vi "抓邊.vi"(0 "Image In":T1, 1 "Process":T7(ring), 2 "Optimized Mode":bool, 3 "Direction":T4(ring), 5 "ROI":T2, 9 "Gap":i32=10 min=1 max=300, 11 "error In":errorcluster, 12 "Edge Options":T5={"Edge Polarity"=0, "Kernel Size"=3, "Width"=3, "Minimum Edge Strength"=10.0, "Interpolation Type"=enum."Bilinear Fixed", "Data Processing Method"=enum."Average"} {"Edge Polarity" items=["All Edges", "Rising Edges", "Falling Edges"]; "Minimum Edge Strength" format="%.2f"; "Width" step=2; "Kernel Size" step=2}, 13 "Point Diameter (5)":u32=5 min=3 max=1000) -> (4 "Image Out":T1, 6 "Line Profile":T3(graph), 10 "Gradient Information":dbl[][](graph), 14 "Line Data":cluster{"X":sgl, "Y":sgl, "T":sgl}, 15 "error out":errorcluster)   [LabVIEW 2015]
uses:
  <vilib>/vision/Measure.llb/Edge Options.ctl
  <vilib>/vision/Measure.llb/Edge Polarity.ctl
  <vilib>/vision/Image Controls.llb/IMAQ Image.ctl
  <vilib>/vision/NI_Vision_Development_Module.lvlib
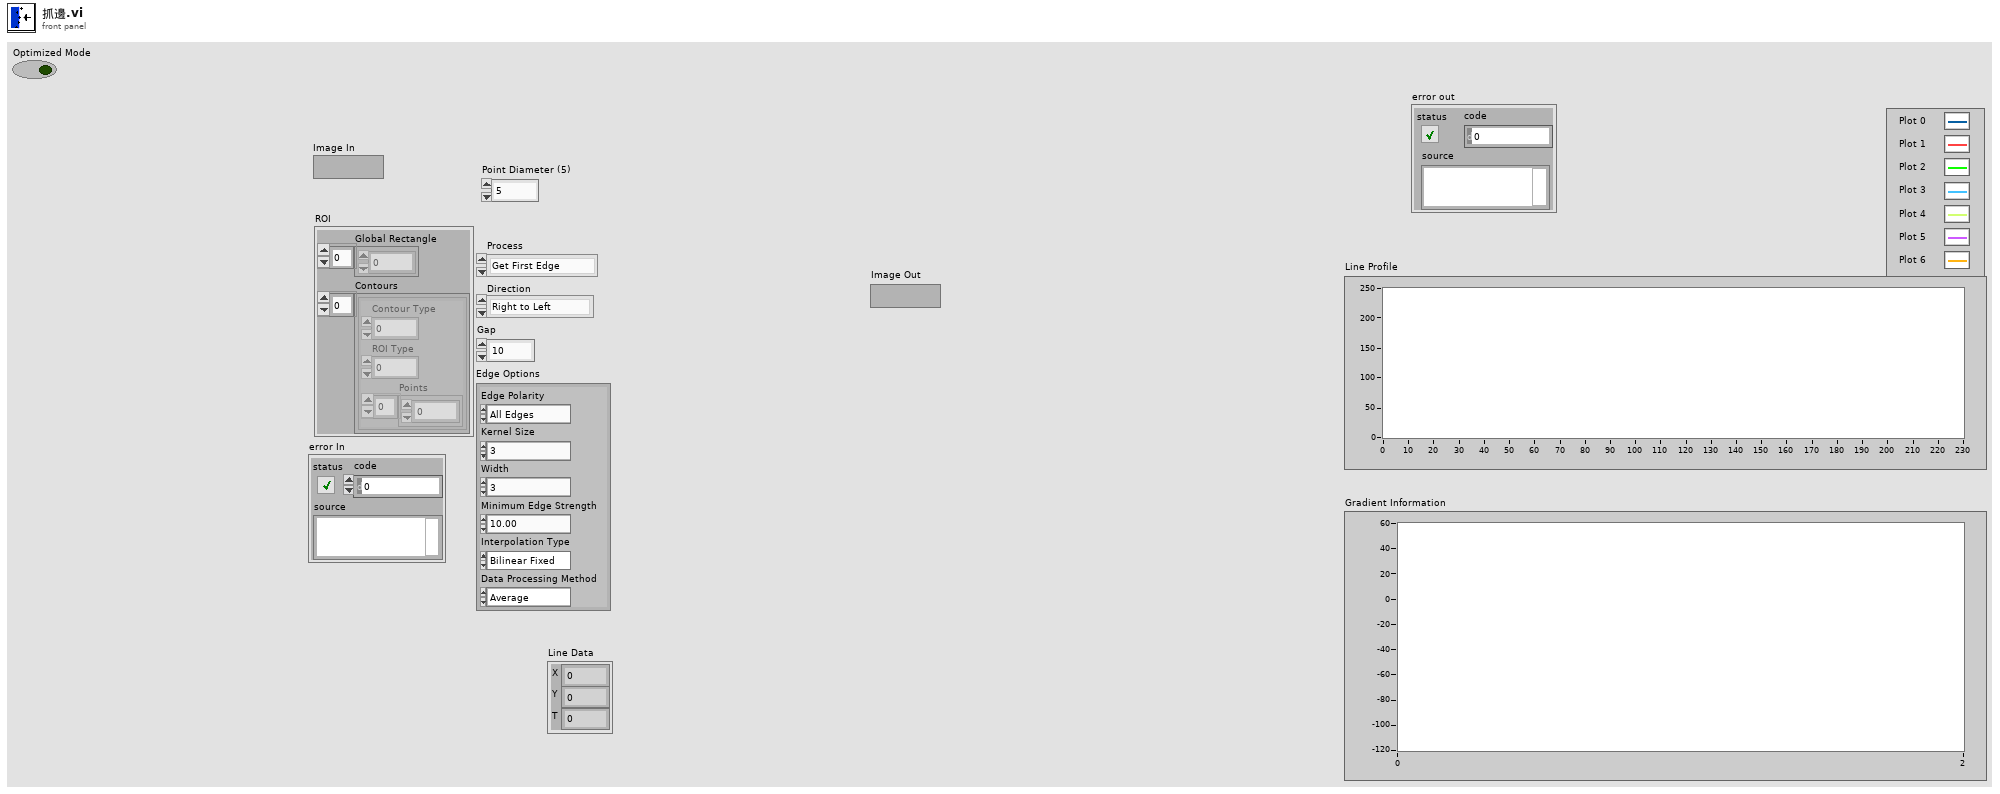
[diagram p1: front panel]
types:
  T1 = typedef "IMAQ Image.ctl" = refnum<image>
  T2 = cluster{"Global Rectangle":i32[], "Contours":cluster{"Contour Type":u32, "ROI Type":u32, "Points":i32[]}[]}
  T3 = cluster{"x0":sgl, "dx":sgl, "Pixels Line":sgl[]}[]
  T4 = enum16{"Right to Left", "Left  to Right", "Up to Down", "Down to Up"}
  T5 = typedef "Edge Options.ctl" = cluster{"Edge Polarity":T6, "Kernel Size":u32, "Width":u32, "Minimum Edge Strength":sgl, "Interpolation Type":enum32{"Zero Order", "Bilinear", "Quadratic", "Cubic", "Bilinear Fixed"}, "Data Processing Method":enum32{"Average", "Median"}}
  T6 = typedef "Edge Polarity.ctl" = u32
  T7 = enum16{"Get First Edge", "Get First + Last Edge", "Get All Edges", "Get Best Edge"}
  T8 = typedef "IMAQ Rectangle" = cluster{"Left":i32, "Top":i32, "Right":i32, "Bottom":i32, "Rotation":dbl}
  T9 = typedef "IMAQ Point" = cluster{"X":sgl, "Y":sgl}
  T10 = cluster{"Point 1":cluster{"x":dbl, "y":dbl}, "Point 2":cluster{"x":dbl, "y":dbl}}
  T11 = typedef "IMAQ Line" = cluster{"Start X":i32, "Start Y":i32, "End X":i32, "End Y":i32}
  T12 = typedef "ROI Descriptor" = cluster{"Global Rectangle":i32[], "Contours":cluster{"ID":enum32{"External", "Internal"}, "Type":u32, "Coordinates":i32[]}[]}
  T13 = typedef "Edge New.ctl" = cluster{"Location (Pixel)":cluster{"X":sgl, "Y":sgl}, "Location (Real-World)":cluster{"X":sgl, "Y":sgl}, "Distance (Pixel)":dbl, "Distance (Real-World)":dbl, "Strength":dbl, "Noise":dbl, "Rising?":bool}
  T14 = cluster{"Point 1":cluster{"X":sgl, "Y":sgl}, "Point 2":cluster{"X":sgl, "Y":sgl}}
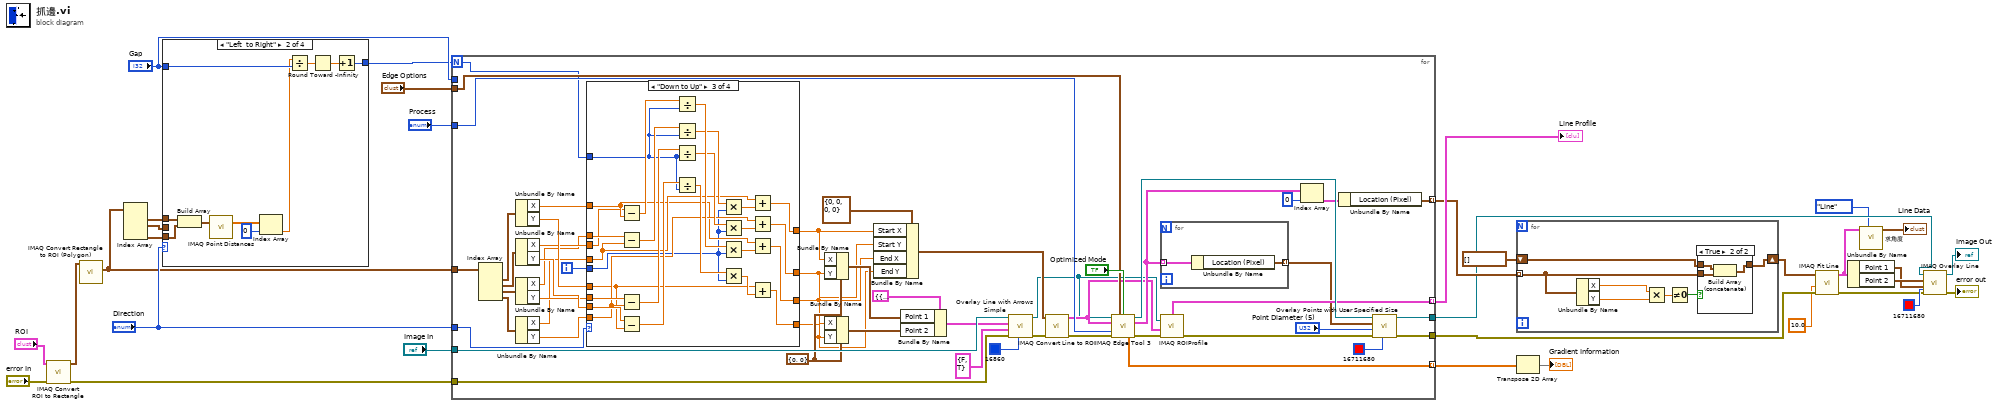
[diagram p0: block diagram]
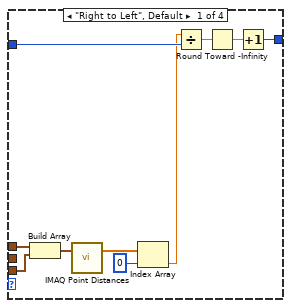
[diagram p2: hidden frame]
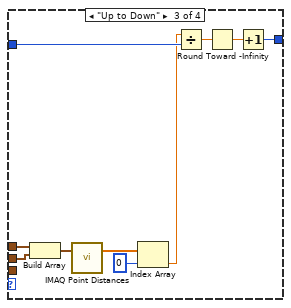
[diagram p3: hidden frame]
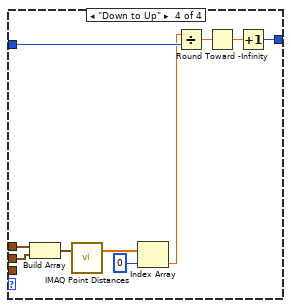
[diagram p4: hidden frame]
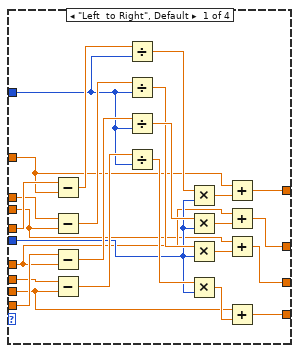
[diagram p6: hidden frame]
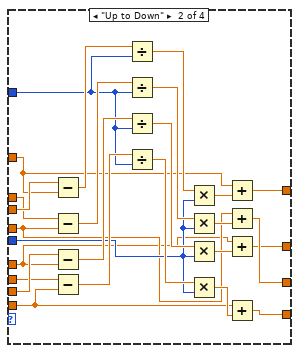
[diagram p7: hidden frame]
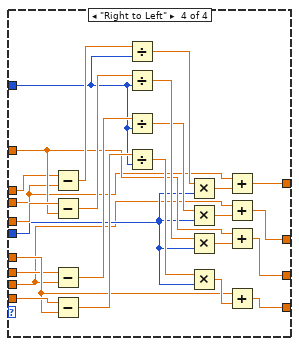
[diagram p8: hidden frame]
diagram:
  n1 = call "IMAQ Convert ROI to Rectangle"("error in (no error)"="error In", "ROI Descriptor"="ROI") -> ("error out"=w24:errorcluster, "Rectangle"=w12:T8)  [unwired: 7 in]
  n2 = call "IMAQ Convert Rectangle to ROI (Polygon)"("Rectangle"=w12) -> ("Rectangle Points"=w18:T9[])  [unwired: 7 in, 2 out]
  n3 = Index Array(array=w18) -> (element #1=w15:T9, element #2=w14:T9, element #4=w13:T9)  [unwired: 4 in, 1 out]
  n4 = case shown="\"Left  to Right\"" "Direction" {
    tunnel: "Gap" -> [w40 w50 w60 w70]
    tunnel: [w39 w49 w59 w69] -> w25
    tunnel: w15 -> [w36 w46 w58 w66]
    tunnel: w13 -> [w35 w45 _ _]
    tunnel: w14 -> [_ _ w54 w65]
    frame "Right to Left", Default {
      n5 = Build Array(w36, w35) -> (w38:T9[])
      n6 = call "IMAQ Point Distances"("Points"=w38) -> ("Distances"=w37:sgl[])  [unwired: 4 in, 1 out]
      n7 = Index Array(array=w37, index=0) -> (element=w33:sgl)
      n8 = Divide(x=w33, y=w40) -> (x/y=w41:sgl)
      n9 = Round Toward -Infinity(1:w41) -> (0:w42:sgl)
      n10 = Increment(x=w42) -> (x+1=w39:i32)
    }
    frame "Left  to Right" {
      n11 = Build Array(w46, w45) -> (w48:T9[])
      n12 = call "IMAQ Point Distances"("Points"=w48) -> ("Distances"=w47:sgl[])  [unwired: 4 in, 1 out]
      n13 = Index Array(array=w47, index=0) -> (element=w43:sgl)
      n14 = Divide(x=w43, y=w50) -> (x/y=w51:sgl)
      n15 = Round Toward -Infinity(1:w51) -> (0:w52:sgl)
      n16 = Increment(x=w52) -> (x+1=w49:i32)
    }
    frame "Up to Down" {
      n17 = Build Array(w58, w54) -> (w57:T9[])
      n18 = call "IMAQ Point Distances"("Points"=w57) -> ("Distances"=w56:sgl[])  [unwired: 4 in, 1 out]
      n19 = Index Array(array=w56, index=0) -> (element=w55:sgl)
      n20 = Divide(x=w55, y=w60) -> (x/y=w61:sgl)
      n21 = Round Toward -Infinity(1:w61) -> (0:w62:sgl)
      n22 = Increment(x=w62) -> (x+1=w59:i32)
    }
    frame "Down to Up" {
      n23 = Build Array(w66, w65) -> (w68:T9[])
      n24 = call "IMAQ Point Distances"("Points"=w68) -> ("Distances"=w67:sgl[])  [unwired: 4 in, 1 out]
      n25 = Index Array(array=w67, index=0) -> (element=w64:sgl)
      n26 = Divide(x=w64, y=w70) -> (x/y=w71:sgl)
      n27 = Round Toward -Infinity(1:w71) -> (0:w72:sgl)
      n28 = Increment(x=w72) -> (x+1=w69:i32)
    }
  }
  n29 = for {
    N: w25 -> [w110]
    tunnel: "Direction" -> [w108]
    tunnel: [w119] -> w21
    tunnel: "Image In" -> [w109]
    tunnel: w24 -> [w106]
    tunnel: [w118] -> w19
    tunnel: "Process" -> [w120]
    tunnel: "Edge Options" -> [w117]
    tunnel: [w116] -> w23 mode=indexing
    tunnel: [w115] -> w26 mode=indexing
    tunnel: [w114] -> w22 mode=indexing
    tunnel: "Gap" -> [_]
    tunnel: w18 -> [w105]
    i -> [w74]
    w102 = cluster{"X":i32, "Y":i32} {"X"=0, "Y"=0} ("Start Point")
    n30 = Index Array(array=w105) -> (element #1=w86:T9, element #2=w85:T9, element #3=w84:T9, element #4=w83:T9)  [unwired: 4 in]
    n31 = Unbundle By Name(w86) -> ("X"=w82:sgl, "Y"=w81:sgl)
    n32 = Unbundle By Name(w85) -> ("X"=w80:sgl, "Y"=w79:sgl)
    n33 = Unbundle By Name(w84) -> ("X"=w78:sgl, "Y"=w77:sgl)
    n34 = Unbundle By Name(w83) -> ("X"=w76:sgl, "Y"=w75:sgl)
    n35 = case shown="\"Down to Up\"" w108 {
      tunnel: [w135 w154 w180 w205] -> w94
      tunnel: [w130 w153 w179 w206] -> w91
      tunnel: [w133 w151 w177 w203] -> w93
      tunnel: [w129 w152 w178 w204] -> w92
      tunnel: w76 -> [w148 w159 w185 w215]
      tunnel: w82 -> [w126 w161 w184 w214]
      tunnel: w110 -> [w139 w163 w190 w216]
      tunnel: w74 -> [w138 w164 w181 w213]
      tunnel: w75 -> [w145 w155 w187 w210]
      tunnel: w81 -> [w128 w157 w186 w209]
      tunnel: w78 -> [w142 w160 w183 w212]
      tunnel: w80 -> [w127 w162 w182 w211]
      tunnel: w77 -> [w137 w156 w188 w208]
      tunnel: w79 -> [w125 w158 w189 w207]
      frame "Left  to Right", Default {
        n36 = Subtract(x=w148, y=w126) -> (x-y=w149:sgl)
        n37 = Subtract(x=w142, y=w127) -> (x-y=w144:sgl)
        n38 = Subtract(x=w145, y=w128) -> (x-y=w147:sgl)
        n39 = Subtract(x=w137, y=w125) -> (x-y=w140:sgl)
        n40 = Divide(x=w149, y=w139) -> (x/y=w150:sgl)
        n41 = Divide(x=w144, y=w139) -> (x/y=w143:sgl)
        n42 = Divide(x=w147, y=w139) -> (x/y=w146:sgl)
        n43 = Divide(x=w140, y=w139) -> (x/y=w141:sgl)
        n44 = Multiply(x=w150, y=w138) -> (x*y=w136:sgl)
        n45 = Multiply(x=w146, y=w138) -> (x*y=w134:sgl)
        n46 = Multiply(x=w143, y=w138) -> (x*y=w132:sgl)
        n47 = Multiply(x=w141, y=w138) -> (x*y=w131:sgl)
        n48 = Add(x=w126, y=w136) -> (x+y=w135:sgl)
        n49 = Add(x=w128, y=w134) -> (x+y=w133:sgl)
        n50 = Add(x=w127, y=w132) -> (x+y=w130:sgl)
        n51 = Add(x=w125, y=w131) -> (x+y=w129:sgl)
      }
      frame "Up to Down" {
        n52 = Subtract(x=w162, y=w161) -> (x-y=w175:sgl)
        n53 = Subtract(x=w160, y=w159) -> (x-y=w172:sgl)
        n54 = Subtract(x=w158, y=w157) -> (x-y=w174:sgl)
        n55 = Subtract(x=w156, y=w155) -> (x-y=w169:sgl)
        n56 = Divide(x=w175, y=w163) -> (x/y=w176:sgl)
        n57 = Divide(x=w172, y=w163) -> (x/y=w171:sgl)
        n58 = Divide(x=w174, y=w163) -> (x/y=w173:sgl)
        n59 = Divide(x=w169, y=w163) -> (x/y=w170:sgl)
        n60 = Multiply(x=w176, y=w164) -> (x*y=w168:sgl)
        n61 = Multiply(x=w171, y=w164) -> (x*y=w166:sgl)
        n62 = Multiply(x=w173, y=w164) -> (x*y=w167:sgl)
        n63 = Multiply(x=w170, y=w164) -> (x*y=w165:sgl)
        n64 = Add(x=w161, y=w168) -> (x+y=w154:sgl)
        n65 = Add(x=w159, y=w166) -> (x+y=w153:sgl)
        n66 = Add(x=w157, y=w167) -> (x+y=w151:sgl)
        n67 = Add(x=w155, y=w165) -> (x+y=w152:sgl)
      }
      frame "Down to Up" {
        n68 = Subtract(x=w182, y=w184) -> (x-y=w201:sgl)
        n69 = Subtract(x=w183, y=w185) -> (x-y=w198:sgl)
        n70 = Subtract(x=w188, y=w187) -> (x-y=w195:sgl)
        n71 = Subtract(x=w189, y=w186) -> (x-y=w200:sgl)
        n72 = Divide(x=w201, y=w190) -> (x/y=w202:sgl)
        n73 = Divide(x=w198, y=w190) -> (x/y=w197:sgl)
        n74 = Divide(x=w195, y=w190) -> (x/y=w196:sgl)
        n75 = Divide(x=w200, y=w190) -> (x/y=w199:sgl)
        n76 = Multiply(x=w197, y=w181) -> (x*y=w192:sgl)
        n77 = Multiply(x=w196, y=w181) -> (x*y=w191:sgl)
        n78 = Multiply(x=w202, y=w181) -> (x*y=w194:sgl)
        n79 = Multiply(x=w199, y=w181) -> (x*y=w193:sgl)
        n80 = Add(x=w185, y=w192) -> (x+y=w180:sgl)
        n81 = Add(x=w187, y=w191) -> (x+y=w177:sgl)
        n82 = Add(x=w184, y=w194) -> (x+y=w179:sgl)
        n83 = Add(x=w186, y=w193) -> (x+y=w178:sgl)
      }
      frame "Right to Left" {
        n84 = Subtract(x=w212, y=w211) -> (x-y=w224:sgl)
        n85 = Subtract(x=w215, y=w214) -> (x-y=w227:sgl)
        n86 = Subtract(x=w208, y=w207) -> (x-y=w221:sgl)
        n87 = Subtract(x=w210, y=w209) -> (x-y=w226:sgl)
        n88 = Divide(x=w224, y=w216) -> (x/y=w223:sgl)
        n89 = Divide(x=w227, y=w216) -> (x/y=w228:sgl)
        n90 = Divide(x=w221, y=w216) -> (x/y=w222:sgl)
        n91 = Divide(x=w226, y=w216) -> (x/y=w225:sgl)
        n92 = Multiply(x=w223, y=w213) -> (x*y=w218:sgl)
        n93 = Multiply(x=w222, y=w213) -> (x*y=w217:sgl)
        n94 = Multiply(x=w228, y=w213) -> (x*y=w220:sgl)
        n95 = Multiply(x=w225, y=w213) -> (x*y=w219:sgl)
        n96 = Add(x=w211, y=w218) -> (x+y=w205:sgl)
        n97 = Add(x=w207, y=w217) -> (x+y=w203:sgl)
        n98 = Add(x=w214, y=w220) -> (x+y=w206:sgl)
        n99 = Add(x=w209, y=w219) -> (x+y=w204:sgl)
      }
    }
    n100 = Bundle By Name(cluster=w102, "X"=w94, "Y"=w93) -> (w100:cluster{"X":i32, "Y":i32})
    n101 = Bundle By Name(cluster=w102, "X"=w91, "Y"=w92) -> (w101:cluster{"X":i32, "Y":i32})
    n102 = Bundle By Name(cluster=T11 {"Start X"=0, "Start Y"=0, "End X"=0, "End Y"=0} ("Line"), "Start X"=w94, "Start Y"=w93, "End X"=w91, "End Y"=w92) -> (w103:T11)
    n103 = Bundle By Name(cluster=T10 {"Point 1"={"x"=50.0, "y"=50.0}, "Point 2"={"x"=70.0, "y"=70.0}} ("Line Coordinates"), "Point 1"=w100, "Point 2"=w101) -> (w97:T10)
    n104 = call "Overlay Line with Arrows Simple.vi"("Color"=u32 16860, "error in"=w106, "Arrows"=cluster{"Start point":bool, "End point":bool} {"Start point"=FALSE, "End point"=TRUE}, "Line Coordinates"=w97, "Image In"=w109) -> ("error out"=w95:errorcluster, "Image Out"=w96:T1)  [unwired: 5 in]
    n105 = call "IMAQ Convert Line to ROI"("error in (no error)"=w95, "Line"=w103) -> ("error out"=w112:errorcluster, "ROI Descriptor"=w111:T12)  [unwired: 7 in]
    n106 = call "IMAQ Edge Tool 3"("Image"=w96, "Edge Options"=w117, "Optimized Mode"="Optimized Mode", "ROI Descriptor"=w111, "Process"=w120, "error in (no error)"=w112) -> ("Image (duplicate)"=w121:T1, "Edge Information"=w124:T13[], "Gradient Values"=w115:dbl[], "error out"=w113:errorcluster)  [unwired: 5 in, 1 out]
    n107 = for {
      tunnel: w124 -> [w230] mode=indexing
      tunnel: [w229] -> w87 mode=indexing
      n108 = Unbundle By Name(w230) -> ("Location (Pixel)"=w229:cluster{"X":sgl, "Y":sgl})
    }
    n109 = call "IMAQ ROIProfile"("error in (no error)"=w113, "ROI Descriptor"=w111, "Image"=w96) -> ("error out"=w123:errorcluster, "ROI Graph"=w116:cluster{"x0":sgl, "dx":sgl, "Pixels Line":sgl[]})  [unwired: 1 in, 3 out]
    n110 = Index Array(array=w124, index=0) -> (element=w88:T13)
    n111 = Unbundle By Name(w88) -> ("Location (Pixel)"=w114:cluster{"X":sgl, "Y":sgl})
    n112 = call "Overlay Points with User Specified Size.vi"("Color"=u32 16711680, "error in"=w123, "Point Diameter (5)"="Point Diameter (5)", "Points"=w87, "Image In"=w121) -> ("error out"=w118:errorcluster, "Image Out"=w119:T1)  [unwired: 5 in]
  }
  "Line Profile" <- w23
  n113 = for {
    tunnel: w22 -> [w233] mode=indexing
    shift-right: [w232] -> w20
    shift-left: cluster{"X":sgl, "Y":sgl}[] [] -> [w231]
    n114 = Unbundle By Name(w233) -> ("X"=w237:sgl, "Y"=w236:sgl)
    n115 = Multiply(x=w237, y=w236) -> (x*y=w235:sgl)
    n116 = Not Equal To 0?(x=w235) -> (x != 0?=w234:bool)
    n117 = case shown="True" w234 {
      tunnel: w233 -> [_ w241]
      tunnel: [w238 w240] -> w232
      tunnel: w231 -> [w238 w239]
      frame False {
      }
      frame True {
        n118 = Build Array (concatenate)(w239, w241) -> (w240:cluster{"X":sgl, "Y":sgl}[])
      }
    }
  }
  n119 = Transpose 2D Array(2D array=w26) -> (transposed array=→"Gradient Information":dbl[][])
  n120 = call "IMAQ Fit Line"("error in (no error)"=w19, "Pixel Radius"=sgl 10.0, "Points"=w20) -> ("error out"=w7:errorcluster, "Line Segment"=w3:T14)  [unwired: 3 in, 4 out]
  n121 = Unbundle By Name(w3) -> ("Point 1"=w8:cluster{"X":sgl, "Y":sgl}, "Point 2"=w9:cluster{"X":sgl, "Y":sgl})
  n122 = call "求角度.vi"("Line form"=enum16{"Line", "Two Point"}."Line", "Line"=w3) -> ("Line Data"=→"Line Data":cluster{"X":sgl, "Y":sgl, "T":sgl})  [unwired: 9 in]
  n123 = call "IMAQ Overlay Line"("Color"=u32 16711680, "error in (no error)"=w7, "End Point"=w9, "Start Point"=w8, "Image"=w21) -> ("error out"=→"error out":errorcluster, "Image Out"=→"Image Out":T1)  [unwired: 5 in]
